vi "OP300ZP_Vout.vi"(8 "errin":errorcluster caption="entrée d'erreur (pas d'erreur)", 11 "VISA":refnum<visa-resource-name> caption="Nom de ressource VISA") -> (0 "errout":errorcluster caption="sortie d'erreur", 3 "Vout lissée":dbl)   [LabVIEW 2020]
uses:
  <vilib>/Instr/_visa.llb/VISA Configure Serial Port (Instr).vi
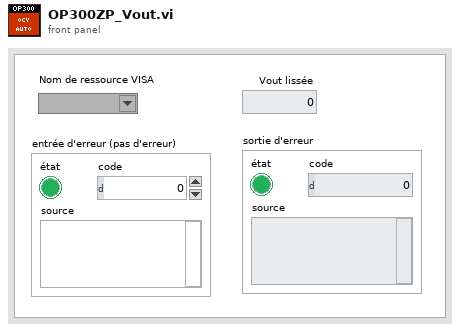
[diagram p1: front panel]
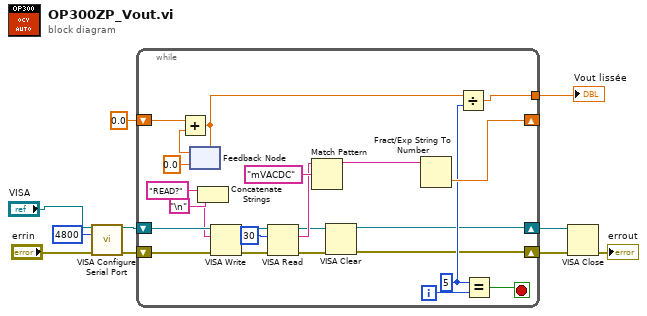
[diagram p0: block diagram]
diagram:
  n1 = call-poly "VISA Configure Serial Port"("VISA resource name"="VISA", "baud rate (9600)"=u32 4800, "error in (no error)"="errin") -> ("VISA resource name out"=w8:refnum<visa-resource-name>, "error out"=w9:errorcluster)  [unwired: 11 in]
  n2 = while {
    shift-right: [w13] -> w6
    shift-left: w9 -> [w34]
    shift-right: [w15] -> w5
    shift-left: w8 -> [w33]
    shift-right: [w22] -> _
    shift-left: 0.0 -> [w21]
    tunnel: [w17] -> w3
    i -> [w23]
    stop <- w24 stop-if-true
    w19 = 5 ("x")
    n3 = feedback #1(0.0) -> (w20:dbl)
    n4 = Add(x=w21, y=w20) -> (x+y=w18:dbl)
    n5 = feedback-in #1(w18) -> ()
    n6 = Concatenate Strings("READ?" ("chaîne"), "\n") -> (w27:string)
    n7 = VISA Write(VISA resource name=w33, write buffer=w27, error in (no error)=w34) -> (VISA resource name out=w29:refnum<visa-resource-name>, error out=w30:errorcluster)  [unwired: 1 out]
    n8 = VISA Read(VISA resource name=w29, byte count=u32 30 ("nombre d'octets"), error in (no error)=w30) -> (VISA resource name out=w16:refnum<visa-resource-name>, read buffer=w25:string, error out=w14:errorcluster)  [unwired: 1 out]
    n9 = Match Pattern(string=w25, regular expression="mVACDC" ("expression régulière")) -> (before substring=w12:string)  [unwired: 1 in, 3 out]
    n10 = VISA Clear(VISA resource name=w16, error in (no error)=w14) -> (VISA resource name out=w15:refnum<visa-resource-name>, error out=w13:errorcluster)
    n11 = Fract/Exp String To Number(string=w12) -> (number=w22:dbl)  [unwired: 3 in, 1 out]
    n12 = Divide(x=w18, y=w19) -> (x/y=w17:dbl)
    n13 = Equal?(x=w19, y=w23) -> (x = y?=w24:bool)
  }
  "Vout lissée" <- w3
  n14 = VISA Close(VISA resource name=w5, error in (no error)=w6) -> (error out=→"errout":errorcluster)
